vi "two_digit_7_segment_display.vi"() -> ()   [LabVIEW 2019]
panel:
  in  "Number":i32
  out "d 2":bool
  out "c 2":bool
  out "e 2":bool
  out "g 2":bool
  out "f 2":bool
  out "b 2":bool
  out "a 2":bool
  out "d":bool
  out "c":bool
  out "e":bool
  out "g":bool
  out "f":bool
  out "b":bool
  out "a":bool
  # "Enter any two digit number to show on the 7-segment display.\nWhen you will enter number more than 2 digits it will show the dialog box."
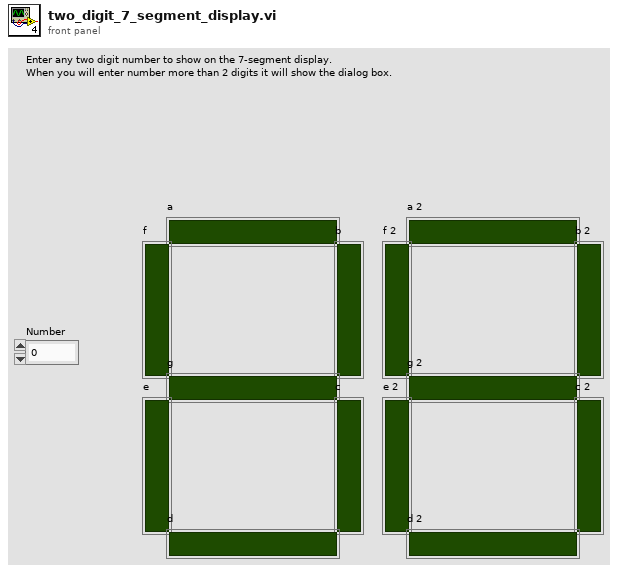
[diagram p1: front panel]
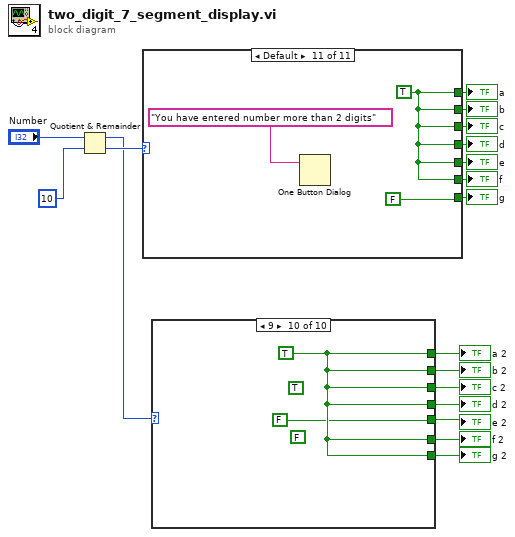
[diagram p0: block diagram]
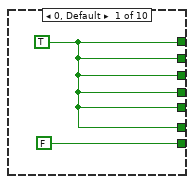
[diagram p2: hidden frame]
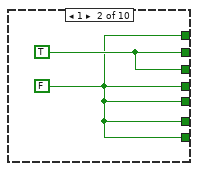
[diagram p3: hidden frame]
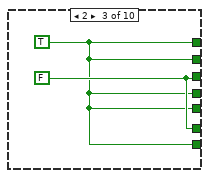
[diagram p4: hidden frame]
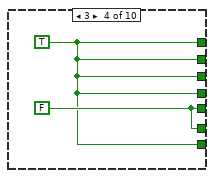
[diagram p5: hidden frame]
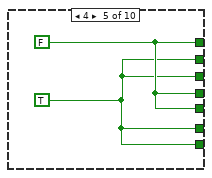
[diagram p6: hidden frame]
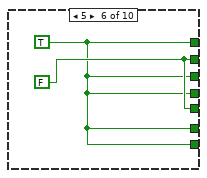
[diagram p7: hidden frame]
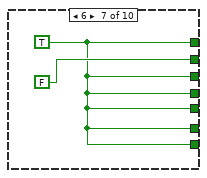
[diagram p8: hidden frame]
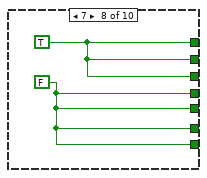
[diagram p9: hidden frame]
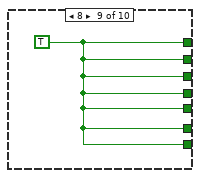
[diagram p10: hidden frame]
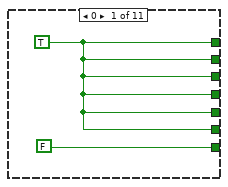
[diagram p11: hidden frame]
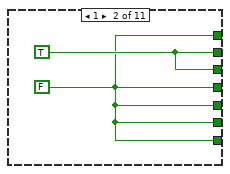
[diagram p12: hidden frame]
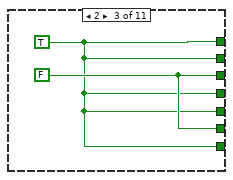
[diagram p13: hidden frame]
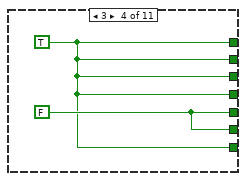
[diagram p14: hidden frame]
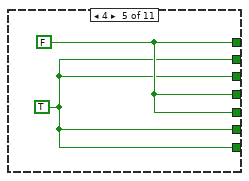
[diagram p15: hidden frame]
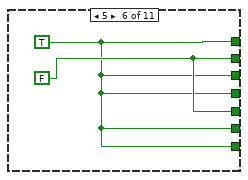
[diagram p16: hidden frame]
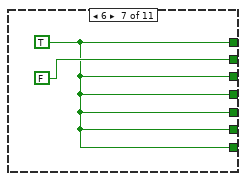
[diagram p17: hidden frame]
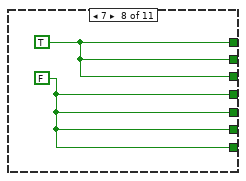
[diagram p18: hidden frame]
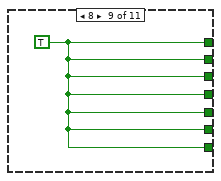
[diagram p19: hidden frame]
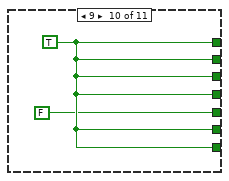
[diagram p20: hidden frame]
diagram:
  (unwired) FALSE
  (unwired) TRUE
  n1 = Quotient & Remainder(x="Number", y=10) -> (x-y*floor(x/y)=w15:i32, floor(x/y)=w16:i32)
  n2 = case shown="Default" w16 {
    tunnel: [w20 w22 w24 w25 w27 w29 w31 w34 w35 w37 w39] -> w14
    tunnel: [w20 w21 w23 w25 w28 w29 w31 w34 w35 w37 w39] -> w13
    tunnel: [w20 w22 w23 w25 w27 w30 FALSE w34 w35 w37 w39] -> w12
    tunnel: [w20 w21 w23 w25 w28 w29 w31 w33 w35 w37 w39] -> w11
    tunnel: [w20 w21 w23 w26 w28 w30 w31 w33 w35 FALSE w39] -> w10
    tunnel: [w20 w21 w24 w26 w27 w29 w31 w33 w35 w37 w39] -> w9
    tunnel: [FALSE w21 w23 w25 w27 w29 w31 w33 w35 w37 FALSE] -> w8
    frame 0 {
      w20 = TRUE
    }
    frame 1 {
      w21 = FALSE
      w22 = TRUE
    }
    frame 2 {
      w24 = FALSE
      w23 = TRUE
    }
    frame 3 {
      w26 = FALSE
      w25 = TRUE
    }
    frame 4 {
      w28 = FALSE
      w27 = TRUE
    }
    frame 5 {
      w30 = FALSE
      w29 = TRUE
    }
    frame 6 {
      w31 = TRUE
    }
    frame 7 {
      w33 = FALSE
      w34 = TRUE
    }
    frame 8 {
      w35 = TRUE
    }
    frame 9 {
      w37 = TRUE
    }
    frame Default {
      w39 = TRUE
      n3 = One Button Dialog(message="You have entered number more than 2 digits") -> ()  [unwired: 1 in, 1 out]
    }
  }
  "a" <- w13
  "b" <- w12
  "f" <- w9
  "g" <- w8
  "e" <- w10
  "c" <- w14
  "d" <- w11
  n4 = case shown="9" w15 {
    tunnel: [w41 w44 w45 w47 w49 w52 FALSE w56 w57 w59] -> w7
    tunnel: [w41 w44 w46 w47 w49 w51 w53 w56 w57 w59] -> w6
    tunnel: [w41 w43 w45 w48 w50 w52 w53 w55 w57 FALSE] -> w5
    tunnel: [w41 w43 w45 w47 w50 w51 w53 w55 w57 w59] -> w4
    tunnel: [w41 w43 w46 w48 w49 w51 w53 w55 w57 w59] -> w3
    tunnel: [FALSE w43 w45 w47 w49 w51 w53 w55 w57 w59] -> w2
    tunnel: [w41 w43 w45 w47 w50 w51 w53 w56 w57 w59] -> w1
    frame 0, Default {
      w41 = TRUE
    }
    frame 1 {
      w43 = FALSE
      w44 = TRUE
    }
    frame 2 {
      w46 = FALSE
      w45 = TRUE
    }
    frame 3 {
      w48 = FALSE
      w47 = TRUE
    }
    frame 4 {
      w49 = TRUE
      w50 = FALSE
    }
    frame 5 {
      w52 = FALSE
      w51 = TRUE
    }
    frame 6 {
      w53 = TRUE
    }
    frame 7 {
      w55 = FALSE
      w56 = TRUE
    }
    frame 8 {
      w57 = TRUE
    }
    frame 9 {
      w59 = TRUE
    }
  }
  "a 2" <- w1
  "b 2" <- w7
  "f 2" <- w3
  "g 2" <- w2
  "e 2" <- w5
  "c 2" <- w6
  "d 2" <- w4
